vi "Read Menu Files.vi"(11 "Measurement Information In":T2={"Comments"="", "Directory Input"="", "Data file path"=path "C:/Data/EPR Data", "Scripting File"=path "C:/Data/Configuration Script.csv", "Save Data"=FALSE, "Tooth size (d11) [mm]"=0.0, "Tooth size (d12) [mm]"=0.0, "Tooth size (d21) [mm]"=0.0, "Tooth size (d22) [mm]"=0.0, "Dose of Tooth [Gy]"=0.0, "Safe Shutdown?"=FALSE, "Gases Available"=[], "Database Username"="", "Database Password"="", "Database Login URL"="", "Database Upload URL"="", "Database Success URL"="", "Database XML URL"="", "Database Resonator URL"="", "Session Number"=0, "Set #"=0, "Resonator Operator"="", "Session Type"="", "Tooth/Sample ID"="", "Volunteer ID"="", "Computer Operator"="", "Volunteer Type"="", "Site/Tooth Selection (T8,T9)"="", "Resonator"="", "Measurement Site"="", "Non-standard session?"=FALSE, "EPR DAQ Version"="", "Session Path"=path "C:/Data/EPR Data", "Chosen Applied State"="", "Chosen Initial State"="", "Time of Transition"="", "DAQ Mode"=enum."Engineering", "pO2/Scan [mmHg]"=[], "pO2/Set [mmHg]"=[], "Linewidth (HWHM)/Scan [Gauss]"=[], "Linewidth (HWHM)/Set [Gauss]"=[], "pO2 Conversion"="", "Dose Calibration Cluster"={"Dose Response"={"grand_mean"=0.0292016, "slope"=0.0188720543}, "Dose Correction"={"Sex"=1, "a0"=7.719669421, "a1"=-2.746550736, "a2"=-0.186490355, "a3"=0.041922063, "a4"=-0.849147359, "a5"=0.14330063, "a6"=0.019930219, "A_n"=40.0, "H_n"=10.12, "Dose Correction"=FALSE}, "Dose Reporting"={"Reporting is"=TRUE, "sd_threshold [AU]"=0.06, "sd_model [Gy]"=0.66, "dosimetric_threshold [Gy]"=2.0, "Add intrasession errors is"=FALSE, "Prior Radiation?"=FALSE}}, "OxyChip Slope"=0.0, "OxyChip Intercept"=0.0, "QA Mode"=enum."Select QA Mode", "QA Session?"=FALSE, "Sample Type"=enum."Empty Resonator", "Report pO2/Scan"=FALSE, "Skip End Session Save"=FALSE, "Number of sites"=enum."# Probes", "Recipient Name"="", "Sender Name"="", "Recipient Email"="", "Transition State History"=[], "pO2 Report Times"=[], "Temperature [C]"=0.0, "+Error pO2/Scan [mmHg]"=[], "-Error pO2/Scan [mmHg]"=[], "+Error pO2/Set [mmHg]"=[], "-Error pO2/Set [mmHg]"=[], "Oxy Phase Exclusion Tolerance [rad]"=0.0, "Oxy Center Exclusion Tolerance [%]"=0.0, "Oxy Exclude Unacceptable"=FALSE, "Oxy Unacceptable Estimate Flags"=[], "Save Session PPT"=FALSE, "Flagged Bad Sets"=[]} {"Oxy Center Exclusion Tolerance [%]" format="%#_9g"; "Oxy Phase Exclusion Tolerance [rad]" format="%#_9g"; "Temperature [C]" format="%#_9g"; "OxyChip Intercept" format="%#_9g"; "OxyChip Slope" format="%#_9g"; "Dose Calibration Cluster"."Dose Reporting"."dosimetric_threshold [Gy]" format="%#_9g"; "Dose Calibration Cluster"."Dose Reporting"."sd_model [Gy]" format="%#_9g"; "Dose Calibration Cluster"."Dose Reporting"."sd_threshold [AU]" format="%#_9g"; "Dose Calibration Cluster"."Dose Correction"."H_n" format="%#_9g"; "Dose Calibration Cluster"."Dose Correction"."A_n" format="%#_9g"; "Dose Calibration Cluster"."Dose Correction"."a6" format="%#.9g"; "Dose Calibration Cluster"."Dose Correction"."a5" format="%#.9g"; "Dose Calibration Cluster"."Dose Correction"."a4" format="%#.9g"; "Dose Calibration Cluster"."Dose Correction"."a3" format="%#.9g"; "Dose Calibration Cluster"."Dose Correction"."a2" format="%#.9g"; "Dose Calibration Cluster"."Dose Correction"."a1" format="%#.9g"; "Dose Calibration Cluster"."Dose Correction"."a0" format="%#.9g"; "Dose Calibration Cluster"."Dose Correction"."Sex" items=["Male"=1, "Female"=0]; "Dose Calibration Cluster"."Dose Response"."slope" format="%#_9g"; "Dose Calibration Cluster"."Dose Response"."grand_mean" format="%#_9g"}) -> (3 "Menu Selections Output":T1)   [LabVIEW 2016]
uses:
  Types/Measurement Information.ctl
  Analysis/Dose Calculation and Reporting/Dose Calculation Control.ctl
  Types/Sample Type.ctl
  <vilib>/Utility/error.llb/whitespace.ctl
panel:
  in  "Menu Selections":T1
  # "Session Information"
  # "Oximetric Data and Information"
  # "Email"
  # "Tooth Information"
  # "Database"
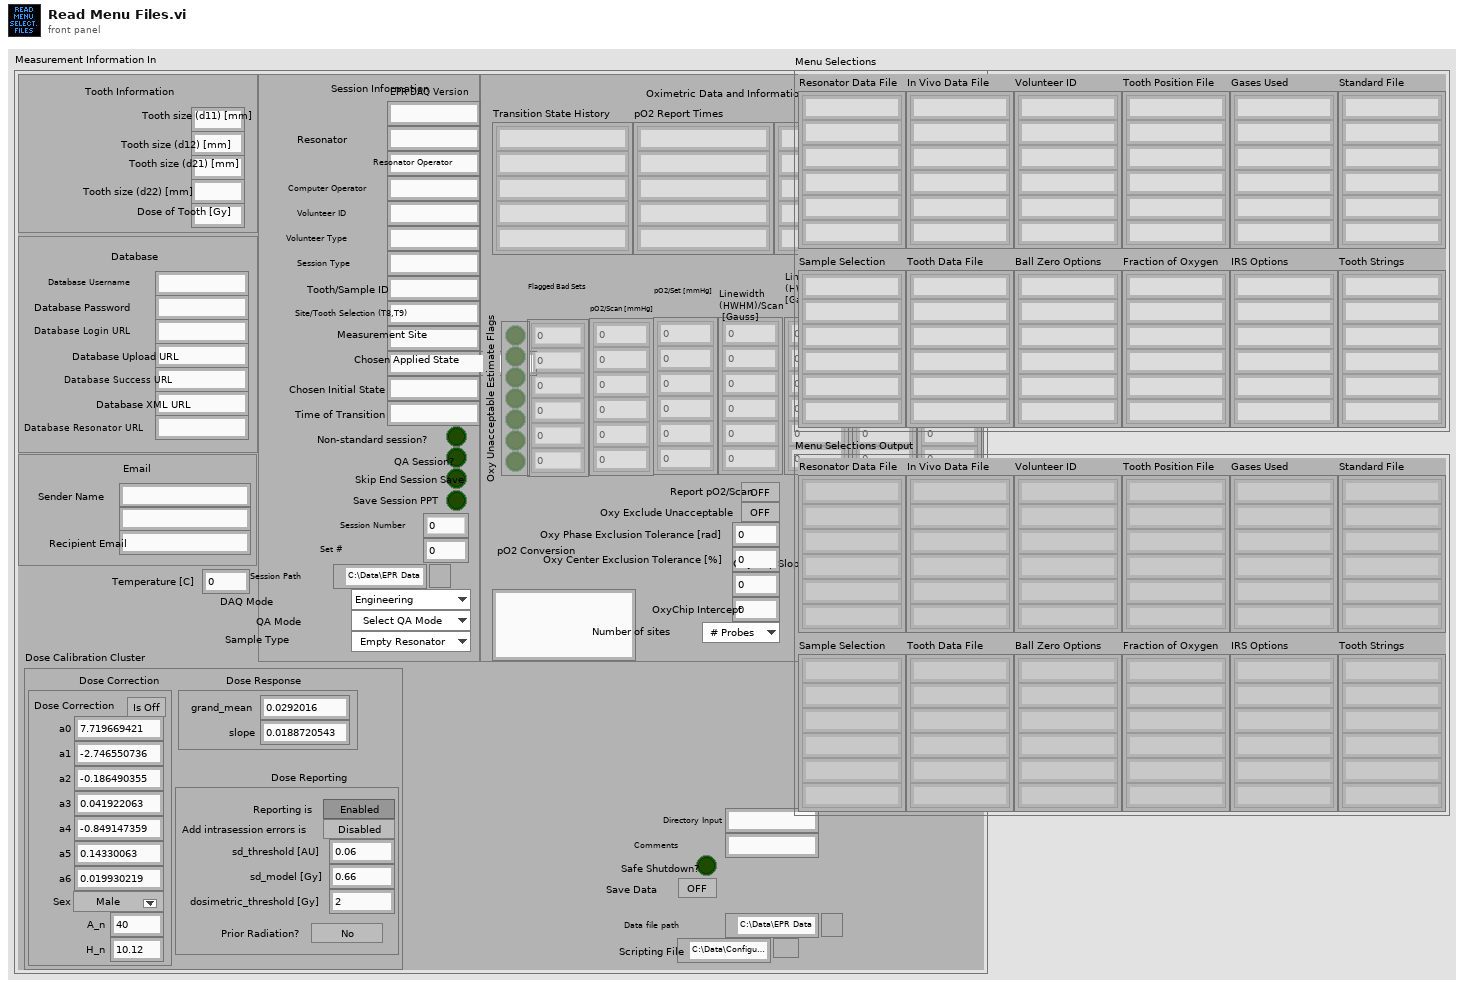
[diagram p1: front panel]
types:
  T1 = cluster{"Resonator Data File":string[], "In Vivo Data File":string[], "Volunteer ID":string[], "Tooth Position File":string[], "Sample Selection":string[], "Tooth Data File":string[], "Ball Zero Options":string[], "Fraction of Oxygen":string[], "Gases Used":string[], "IRS Options":string[], "Standard File":string[], "Tooth Strings":string[]}
  T2 = typedef "Measurement Information.ctl" = cluster{"Comments":string, "Directory Input":string, "Data file path":path, "Scripting File":path, "Save Data":bool, "Tooth size (d11) [mm]":dbl, "Tooth size (d12) [mm]":dbl, "Tooth size (d21) [mm]":dbl, "Tooth size (d22) [mm]":dbl, "Dose of Tooth [Gy]":dbl, "Safe Shutdown?":bool, "Gases Available":string[], "Database Username":string, "Database Password":string, "Database Login URL":string, "Database Upload URL":string, "Database Success URL":string, "Database XML URL":string, "Database Resonator URL":string, "Session Number":i32, "Set #":u32, "Resonator Operator":string, "Session Type":string, "Tooth/Sample ID":string, "Volunteer ID":string, "Computer Operator":string, "Volunteer Type":string, "Site/Tooth Selection (T8,T9)":string, "Resonator":string, "Measurement Site":string, "Non-standard session?":bool, "EPR DAQ Version":string, "Session Path":path, "Chosen Applied State":string, "Chosen Initial State":string, "Time of Transition":string, "DAQ Mode":enum16{"Engineering", "Dosimetry", "Oximetry"}, "pO2/Scan [mmHg]":dbl[][], "pO2/Set [mmHg]":dbl[][], "Linewidth (HWHM)/Scan [Gauss]":dbl[][], "Linewidth (HWHM)/Set [Gauss]":dbl[][], "pO2 Conversion":string, "Dose Calibration Cluster":T3, "OxyChip Slope":dbl, "OxyChip Intercept":dbl, "QA Mode":enum16{"Select QA Mode", "QA-Start/End", "QA-Mid", "QA-Weekly", "QA-Eng", "Check Calibration"}, "QA Session?":bool, "Sample Type":T4, "Report pO2/Scan":bool, "Skip End Session Save":bool, "Number of sites":enum16{"# Probes", "1", "2", "3", "4"}, "Recipient Name":string, "Sender Name":string, "Recipient Email":string, "Transition State History":string[], "pO2 Report Times":string[], "Temperature [C]":dbl, "+Error pO2/Scan [mmHg]":dbl[][], "-Error pO2/Scan [mmHg]":dbl[][], "+Error pO2/Set [mmHg]":dbl[][], "-Error pO2/Set [mmHg]":dbl[][], "Oxy Phase Exclusion Tolerance [rad]":dbl, "Oxy Center Exclusion Tolerance [%]":dbl, "Oxy Exclude Unacceptable":bool, "Oxy Unacceptable Estimate Flags":bool[], "Save Session PPT":bool, "Flagged Bad Sets":u32[]}
  T3 = typedef "Dose Calculation Control.ctl" = cluster{"Dose Response":cluster{"grand_mean":dbl, "slope":dbl}, "Dose Correction":cluster{"Sex":u16, "a0":dbl, "a1":dbl, "a2":dbl, "a3":dbl, "a4":dbl, "a5":dbl, "a6":dbl, "A_n":dbl, "H_n":dbl, "Dose Correction":bool}, "Dose Reporting":cluster{"Reporting is":bool, "sd_threshold [AU]":dbl, "sd_model [Gy]":dbl, "dosimetric_threshold [Gy]":dbl, "Add intrasession errors is":bool, "Prior Radiation?":bool}}
  T4 = typedef "Sample Type.ctl" = enum16{"Empty Resonator", "IRS", "BallZero", "Irradiated Tooth", "Non-irradiated Tooth", "OxyChip", "LiPc", "PDT", "India Ink"}
  T5 = typedef "whitespace.ctl" = u16
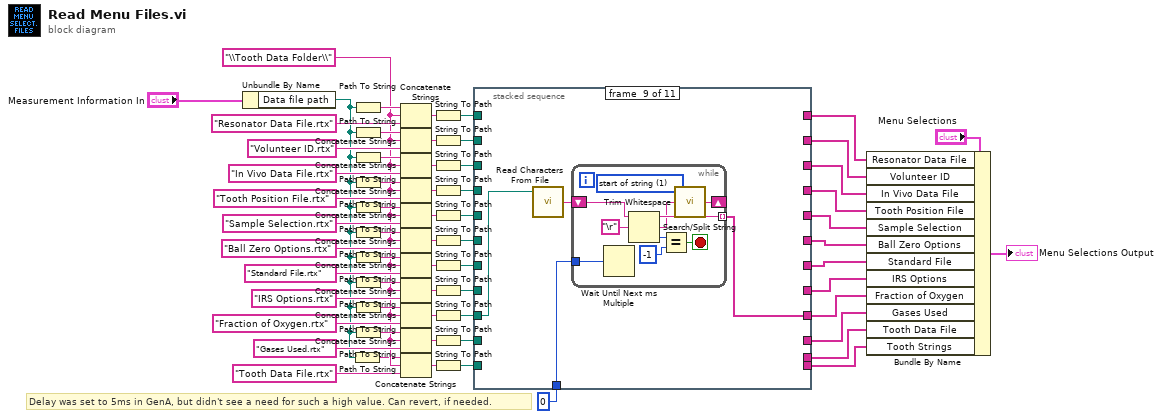
[diagram p0: block diagram]
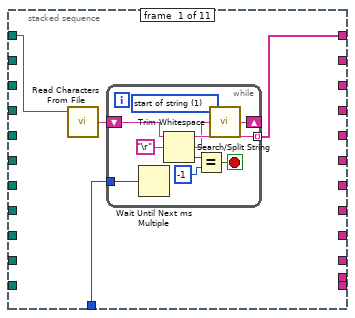
[diagram p2: hidden frame]
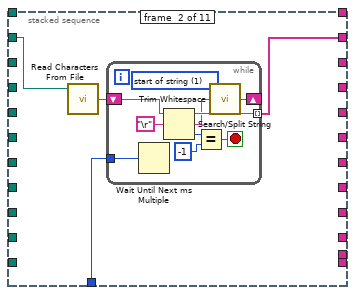
[diagram p3: hidden frame]
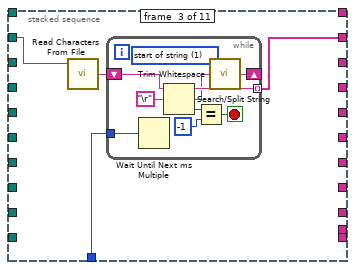
[diagram p4: hidden frame]
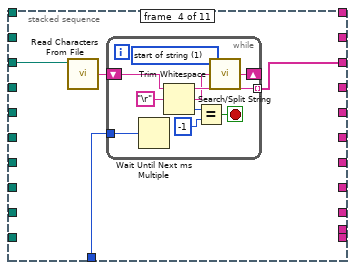
[diagram p5: hidden frame]
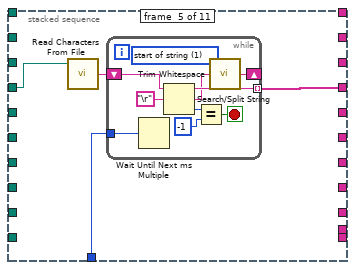
[diagram p6: hidden frame]
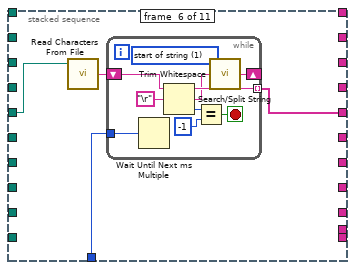
[diagram p7: hidden frame]
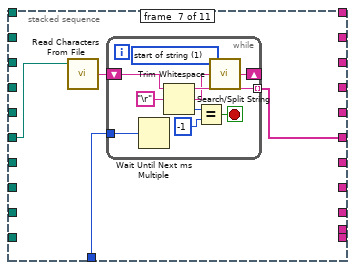
[diagram p8: hidden frame]
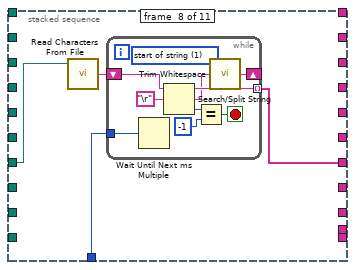
[diagram p9: hidden frame]
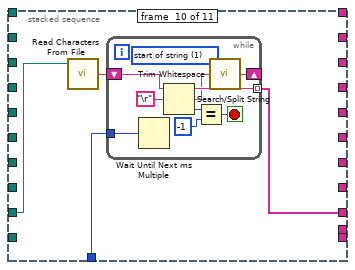
[diagram p10: hidden frame]
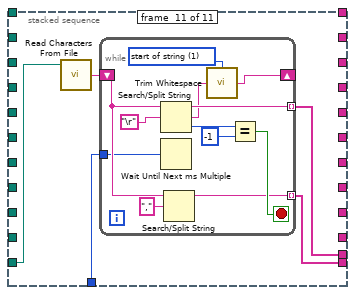
[diagram p11: hidden frame]
diagram:
  w19 = "\\Tooth Data Folder\\" ("string")
  # "Delay was set to 5ms in GenA, but didn't see a need for such a high value. Can revert, if needed."
  n1 = Unbundle By Name("Measurement Information In") -> ("Data file path"=w20:path)
  n2 = Path To String(path=w20) -> (string=w18:string)
  n3 = Path To String(path=w20) -> (string=w61:string)
  n4 = Path To String(path=w20) -> (string=w52:string)
  n5 = Path To String(path=w20) -> (string=w58:string)
  n6 = Path To String(path=w20) -> (string=w56:string)
  n7 = Path To String(path=w20) -> (string=w46:string)
  n8 = Path To String(path=w20) -> (string=w38:string)
  n9 = Path To String(path=w20) -> (string=w37:string)
  n10 = Path To String(path=w20) -> (string=w32:string)
  n11 = Path To String(path=w20) -> (string=w49:string)
  n12 = Path To String(path=w20) -> (string=w43:string)
  n13 = Concatenate Strings(w61, w19, "Resonator Data File.rtx" ("string")) -> (w60:string)
  n14 = Concatenate Strings(w52, w19, "Volunteer ID.rtx" ("string")) -> (w51:string)
  n15 = Concatenate Strings(w58, w19, "In Vivo Data File.rtx" ("string")) -> (w57:string)
  n16 = Concatenate Strings(w56, w19, "Tooth Position File.rtx" ("string")) -> (w55:string)
  n17 = Concatenate Strings(w46, w19, "Sample Selection.rtx" ("string")) -> (w45:string)
  n18 = Concatenate Strings(w38, w19, "Ball Zero Options.rtx" ("string")) -> (w39:string)
  n19 = Concatenate Strings(w37, w19, "Standard File.rtx" ("string")) -> (w36:string)
  n20 = Concatenate Strings(w32, w19, "IRS Options.rtx" ("string")) -> (w33:string)
  n21 = Concatenate Strings(w49, w19, "Fraction of Oxygen.rtx" ("string")) -> (w48:string)
  n22 = Concatenate Strings(w43, w19, "Gases Used.rtx" ("string")) -> (w42:string)
  n23 = Concatenate Strings(w18, w19, "Tooth Data File.rtx" ("string")) -> (w21:string)
  n24 = String To Path(string=w60) -> (path=w31:path)
  n25 = String To Path(string=w51) -> (path=w30:path)
  n26 = String To Path(string=w57) -> (path=w29:path)
  n27 = String To Path(string=w55) -> (path=w28:path)
  n28 = String To Path(string=w45) -> (path=w27:path)
  n29 = String To Path(string=w39) -> (path=w26:path)
  n30 = String To Path(string=w36) -> (path=w25:path)
  n31 = String To Path(string=w33) -> (path=w24:path)
  n32 = String To Path(string=w48) -> (path=w23:path)
  n33 = String To Path(string=w42) -> (path=w22:path)
  n34 = String To Path(string=w21) -> (path=w16:path)
  n35 = stacked-sequence {
    tunnel: w31 -> [w65 _ _ _ _ _ _ _ _ _ _]
    tunnel: w30 -> [_ w79 _ _ _ _ _ _ _ _ _]
    tunnel: w29 -> [_ _ w93 _ _ _ _ _ _ _ _]
    tunnel: w28 -> [_ _ _ w107 _ _ _ _ _ _ _]
    tunnel: w27 -> [_ _ _ _ w121 _ _ _ _ _ _]
    tunnel: w26 -> [_ _ _ _ _ w135 _ _ _ _ _]
    tunnel: w25 -> [_ _ _ _ _ _ w149 _ _ _ _]
    tunnel: w24 -> [_ _ _ _ _ _ _ w163 _ _ _]
    tunnel: w23 -> [_ _ _ _ _ _ _ _ w177 _ _]
    tunnel: w22 -> [_ _ _ _ _ _ _ _ _ w191 _]
    tunnel: [w64 _ _ _ _ _ _ _ _ _ _] -> w14
    tunnel: [_ w78 _ _ _ _ _ _ _ _ _] -> w12
    tunnel: w16 -> [_ _ _ _ _ _ _ _ _ _ w206]
    tunnel: [_ _ _ _ _ _ _ _ _ _ w205] -> w3
    tunnel: [_ _ _ _ _ _ _ _ _ _ w204] -> w2
    tunnel: [_ _ w92 _ _ _ _ _ _ _ _] -> w11
    tunnel: [_ _ _ w106 _ _ _ _ _ _ _] -> w10
    tunnel: [_ _ _ _ w120 _ _ _ _ _ _] -> w9
    tunnel: [_ _ _ _ _ w134 _ _ _ _ _] -> w8
    tunnel: [_ _ _ _ _ _ w148 _ _ _ _] -> w7
    tunnel: [_ _ _ _ _ _ _ w162 _ _ _] -> w6
    tunnel: [_ _ _ _ _ _ _ _ w176 _ _] -> w5
    tunnel: [_ _ _ _ _ _ _ _ _ w190 _] -> w4
    tunnel: u32 0 ("millisecond multiple") -> [w63 w77 w91 w105 w119 w133 w147 w161 w175 w189 w203]
    frame #0 {
      n36 = call <vilib>:"Read Characters From File.vi"("file path (dialog if empty)"=w65) -> ("character string"=w66:string)  [unwired: 1 in, 7 out]
      n37 = while {
        shift-right: [w72] -> _
        shift-left: w66 -> [w76]
        tunnel: [w75] -> w64 mode=indexing
        tunnel: w63 -> [w67]
        stop <- w69 stop-if-true
        w73 = T5 1 items=["both", "start of string", "end of string"] ("location (both)")
        n38 = Wait Until Next ms Multiple(millisecond multiple=w67) -> ()  [unwired: 1 out]
        n39 = Search/Split String(string=w76, search string/char (-)="\r") -> (substring before match=w75:string, match + rest of string=w74:string, offset of match=w71:i32)  [unwired: 1 out]
        n40 = Equal?(x=w71, y=-1) -> (x = y?=w69:bool)
        n41 = call <vilib>:"Trim Whitespace.vi"("string"=w74, "location (both)"=w73) -> ("trimmed string"=w72:string)
      }
    }
    frame #1 {
      n42 = call <vilib>:"Read Characters From File.vi"("file path (dialog if empty)"=w79) -> ("character string"=w80:string)  [unwired: 1 in, 7 out]
      n43 = while {
        shift-right: [w86] -> _
        shift-left: w80 -> [w90]
        tunnel: [w89] -> w78 mode=indexing
        tunnel: w77 -> [w81]
        stop <- w83 stop-if-true
        w87 = T5 1 items=["both", "start of string", "end of string"] ("location (both)")
        n44 = Wait Until Next ms Multiple(millisecond multiple=w81) -> ()  [unwired: 1 out]
        n45 = Search/Split String(string=w90, search string/char (-)="\r") -> (substring before match=w89:string, match + rest of string=w88:string, offset of match=w85:i32)  [unwired: 1 out]
        n46 = Equal?(x=w85, y=-1) -> (x = y?=w83:bool)
        n47 = call <vilib>:"Trim Whitespace.vi"("string"=w88, "location (both)"=w87) -> ("trimmed string"=w86:string)
      }
    }
    frame #2 {
      n48 = call <vilib>:"Read Characters From File.vi"("file path (dialog if empty)"=w93) -> ("character string"=w94:string)  [unwired: 1 in, 7 out]
      n49 = while {
        shift-right: [w100] -> _
        shift-left: w94 -> [w104]
        tunnel: [w103] -> w92 mode=indexing
        tunnel: w91 -> [w95]
        stop <- w97 stop-if-true
        w101 = T5 1 items=["both", "start of string", "end of string"] ("location (both)")
        n50 = Wait Until Next ms Multiple(millisecond multiple=w95) -> ()  [unwired: 1 out]
        n51 = Search/Split String(string=w104, search string/char (-)="\r") -> (substring before match=w103:string, match + rest of string=w102:string, offset of match=w99:i32)  [unwired: 1 out]
        n52 = Equal?(x=w99, y=-1) -> (x = y?=w97:bool)
        n53 = call <vilib>:"Trim Whitespace.vi"("string"=w102, "location (both)"=w101) -> ("trimmed string"=w100:string)
      }
    }
    frame #3 {
      n54 = call <vilib>:"Read Characters From File.vi"("file path (dialog if empty)"=w107) -> ("character string"=w108:string)  [unwired: 1 in, 7 out]
      n55 = while {
        shift-right: [w114] -> _
        shift-left: w108 -> [w118]
        tunnel: [w117] -> w106 mode=indexing
        tunnel: w105 -> [w109]
        stop <- w111 stop-if-true
        w115 = T5 1 items=["both", "start of string", "end of string"] ("location (both)")
        n56 = Wait Until Next ms Multiple(millisecond multiple=w109) -> ()  [unwired: 1 out]
        n57 = Search/Split String(string=w118, search string/char (-)="\r") -> (substring before match=w117:string, match + rest of string=w116:string, offset of match=w113:i32)  [unwired: 1 out]
        n58 = Equal?(x=w113, y=-1) -> (x = y?=w111:bool)
        n59 = call <vilib>:"Trim Whitespace.vi"("string"=w116, "location (both)"=w115) -> ("trimmed string"=w114:string)
      }
    }
    frame #4 {
      n60 = call <vilib>:"Read Characters From File.vi"("file path (dialog if empty)"=w121) -> ("character string"=w122:string)  [unwired: 1 in, 7 out]
      n61 = while {
        shift-right: [w128] -> _
        shift-left: w122 -> [w132]
        tunnel: [w131] -> w120 mode=indexing
        tunnel: w119 -> [w123]
        stop <- w125 stop-if-true
        w129 = T5 1 items=["both", "start of string", "end of string"] ("location (both)")
        n62 = Wait Until Next ms Multiple(millisecond multiple=w123) -> ()  [unwired: 1 out]
        n63 = Search/Split String(string=w132, search string/char (-)="\r") -> (substring before match=w131:string, match + rest of string=w130:string, offset of match=w127:i32)  [unwired: 1 out]
        n64 = Equal?(x=w127, y=-1) -> (x = y?=w125:bool)
        n65 = call <vilib>:"Trim Whitespace.vi"("string"=w130, "location (both)"=w129) -> ("trimmed string"=w128:string)
      }
    }
    frame #5 {
      n66 = call <vilib>:"Read Characters From File.vi"("file path (dialog if empty)"=w135) -> ("character string"=w136:string)  [unwired: 1 in, 7 out]
      n67 = while {
        shift-right: [w142] -> _
        shift-left: w136 -> [w146]
        tunnel: [w145] -> w134 mode=indexing
        tunnel: w133 -> [w137]
        stop <- w139 stop-if-true
        w143 = T5 1 items=["both", "start of string", "end of string"] ("location (both)")
        n68 = Wait Until Next ms Multiple(millisecond multiple=w137) -> ()  [unwired: 1 out]
        n69 = Search/Split String(string=w146, search string/char (-)="\r") -> (substring before match=w145:string, match + rest of string=w144:string, offset of match=w141:i32)  [unwired: 1 out]
        n70 = Equal?(x=w141, y=-1) -> (x = y?=w139:bool)
        n71 = call <vilib>:"Trim Whitespace.vi"("string"=w144, "location (both)"=w143) -> ("trimmed string"=w142:string)
      }
    }
    frame #6 {
      n72 = call <vilib>:"Read Characters From File.vi"("file path (dialog if empty)"=w149) -> ("character string"=w150:string)  [unwired: 1 in, 7 out]
      n73 = while {
        shift-right: [w156] -> _
        shift-left: w150 -> [w160]
        tunnel: [w159] -> w148 mode=indexing
        tunnel: w147 -> [w151]
        stop <- w153 stop-if-true
        w157 = T5 1 items=["both", "start of string", "end of string"] ("location (both)")
        n74 = Wait Until Next ms Multiple(millisecond multiple=w151) -> ()  [unwired: 1 out]
        n75 = Search/Split String(string=w160, search string/char (-)="\r") -> (substring before match=w159:string, match + rest of string=w158:string, offset of match=w155:i32)  [unwired: 1 out]
        n76 = Equal?(x=w155, y=-1) -> (x = y?=w153:bool)
        n77 = call <vilib>:"Trim Whitespace.vi"("string"=w158, "location (both)"=w157) -> ("trimmed string"=w156:string)
      }
    }
    frame #7 {
      n78 = call <vilib>:"Read Characters From File.vi"("file path (dialog if empty)"=w163) -> ("character string"=w164:string)  [unwired: 1 in, 7 out]
      n79 = while {
        shift-right: [w170] -> _
        shift-left: w164 -> [w174]
        tunnel: [w173] -> w162 mode=indexing
        tunnel: w161 -> [w165]
        stop <- w167 stop-if-true
        w171 = T5 1 items=["both", "start of string", "end of string"] ("location (both)")
        n80 = Wait Until Next ms Multiple(millisecond multiple=w165) -> ()  [unwired: 1 out]
        n81 = Search/Split String(string=w174, search string/char (-)="\r") -> (substring before match=w173:string, match + rest of string=w172:string, offset of match=w169:i32)  [unwired: 1 out]
        n82 = Equal?(x=w169, y=-1) -> (x = y?=w167:bool)
        n83 = call <vilib>:"Trim Whitespace.vi"("string"=w172, "location (both)"=w171) -> ("trimmed string"=w170:string)
      }
    }
    frame #8 {
      n84 = call <vilib>:"Read Characters From File.vi"("file path (dialog if empty)"=w177) -> ("character string"=w178:string)  [unwired: 1 in, 7 out]
      n85 = while {
        shift-right: [w184] -> _
        shift-left: w178 -> [w188]
        tunnel: [w187] -> w176 mode=indexing
        tunnel: w175 -> [w179]
        stop <- w181 stop-if-true
        w185 = T5 1 items=["both", "start of string", "end of string"] ("location (both)")
        n86 = Wait Until Next ms Multiple(millisecond multiple=w179) -> ()  [unwired: 1 out]
        n87 = Search/Split String(string=w188, search string/char (-)="\r") -> (substring before match=w187:string, match + rest of string=w186:string, offset of match=w183:i32)  [unwired: 1 out]
        n88 = Equal?(x=w183, y=-1) -> (x = y?=w181:bool)
        n89 = call <vilib>:"Trim Whitespace.vi"("string"=w186, "location (both)"=w185) -> ("trimmed string"=w184:string)
      }
    }
    frame #9 {
      n90 = call <vilib>:"Read Characters From File.vi"("file path (dialog if empty)"=w191) -> ("character string"=w192:string)  [unwired: 1 in, 7 out]
      n91 = while {
        shift-right: [w198] -> _
        shift-left: w192 -> [w202]
        tunnel: [w201] -> w190 mode=indexing
        tunnel: w189 -> [w193]
        stop <- w195 stop-if-true
        w199 = T5 1 items=["both", "start of string", "end of string"] ("location (both)")
        n92 = Wait Until Next ms Multiple(millisecond multiple=w193) -> ()  [unwired: 1 out]
        n93 = Search/Split String(string=w202, search string/char (-)="\r") -> (substring before match=w201:string, match + rest of string=w200:string, offset of match=w197:i32)  [unwired: 1 out]
        n94 = Equal?(x=w197, y=-1) -> (x = y?=w195:bool)
        n95 = call <vilib>:"Trim Whitespace.vi"("string"=w200, "location (both)"=w199) -> ("trimmed string"=w198:string)
      }
    }
    frame #10 {
      n96 = call <vilib>:"Read Characters From File.vi"("file path (dialog if empty)"=w206) -> ("character string"=w207:string)  [unwired: 1 in, 7 out]
      n97 = while {
        shift-right: [w216] -> _
        shift-left: w207 -> [w211]
        tunnel: [w219] -> w205 mode=indexing
        tunnel: [w209] -> w204 mode=indexing
        tunnel: w203 -> [w208]
        stop <- w213 stop-if-true
        w217 = T5 1 items=["both", "start of string", "end of string"] ("location (both)")
        n98 = Search/Split String(string=w211, search string/char (-)="\r") -> (substring before match=w219:string, match + rest of string=w218:string, offset of match=w215:i32)  [unwired: 1 out]
        n99 = Wait Until Next ms Multiple(millisecond multiple=w208) -> ()  [unwired: 1 out]
        n100 = Search/Split String(string=w211, search string/char (-)=",") -> (substring before match=w209:string)  [unwired: 3 out]
        n101 = call <vilib>:"Trim Whitespace.vi"("string"=w218, "location (both)"=w217) -> ("trimmed string"=w216:string)
        n102 = Equal?(x=w215, y=-1) -> (x = y?=w213:bool)
      }
    }
  }
  n103 = Bundle By Name(cluster="Menu Selections", "Resonator Data File"=w14, "Volunteer ID"=w12, "In Vivo Data File"=w11, "Tooth Position File"=w10, "Sample Selection"=w9, "Ball Zero Options"=w8, "Standard File"=w7, "IRS Options"=w6, "Fraction of Oxygen"=w5, "Gases Used"=w4, "Tooth Data File"=w3, "Tooth Strings"=w2) -> (→"Menu Selections Output":T1)
